vi "Diagnostics - Tool.vi"() -> ()   [LabVIEW 2019, in "Diagnostics Workspace Tool.lvlib"]
uses:
  Diagnostics Workspace Tool.lvlib
  Addon/Addon Shared/Types/Command.New.ctl
  NationalInstruments.VeriStand.SystemStorage
  SubModules/CAN-Streaming-Support/Addon/Addon Shared/Types/Direction Filter.ctl
  SubModules/CAN-Streaming-Support/Addon/Addon Shared/Types/Type Filter.ctl
  Workspace Shared/Types/Workspace.State.ctl
  Workspace Shared/Types/UI.Refs.ctl
  <vilib>/NI VeriStand/Display Template Support/DisplayTemplateSupport.llb/enum_Display Template Handler Minimal To Workspace.ctl
  Workspace Shared/Types/Workspace.SavedState.ctl
  <vilib>/NI VeriStand/Execution/Workspace/WorkspaceAPI.ctl
  <vilib>/NI VeriStand/Display Template Support/DisplayTemplateSupport.llb/enum_Display Template Handler Minimal To Widget Msg.ctl
  <vilib>/NI VeriStand/Execution/Workspace/SystemStateRegEventRef.ctl
  <vilib>/NI VeriStand/Execution/Workspace/Target State Info.ctl
  <vilib>/NI VeriStand/Execution/Workspace/Target State.ctl
  <vilib>/NI VeriStand/Execution/Workspace/SystemStateEventRef.ctl
  Addon/Addon Shared/Types/Protocol.ctl
  SubModules/CAN-Streaming-Support/UIs/Workspace Shared/Types/Host Stream Queue Refs.ctl
  SubModules/CAN-Streaming-Support/UIs/Workspace Shared/Types/Host Stream Queue Type.ctl
  SubModules/CAN-Streaming-Support/UIs/Workspace Shared/Types/Host Stream Queue Command.ctl
  <vilib>/xnet/xnet.llb/XNET Frame CAN.ctl
  <vilib>/xnet/xnet.llb/XNET Frame Type CAN.ctl
  SubModules/CAN-Streaming-Support/UIs/Workspace Shared/Types/Host Stream Engine Parameters.ctl
  SubModules/CAN-Streaming-Support/Addon/Addon Shared/Types/Filter Parameters.ctl
  Addon/Addon Shared/Types/Command.ReadDTC.ctl
  Addon/Addon Shared/Types/DTC.Descriptor.Override.ctl
  <vilib>/Utility/miscctls.llb/LVRowAndColumnUnsignedTypeDef.ctl
  <vilib>/dlg_ctls.llb/Space Constant.vi
  SubModules/CAN-Streaming-Support/UIs/Workspace Shared/SubVIs/Create Host Stream Refs.vi
  SubModules/CAN-Streaming-Support/UIs/Workspace Shared/SubVIs/Read Host Stream.vi
  SubModules/CAN-Streaming-Support/UIs/Workspace Shared/SubVIs/Cleanup Host Stream.vi
  SubModules/CAN-Streaming-Support/UIs/Workspace Shared/SubVIs/Create Bus Log File.vi
  SubModules/CAN-Streaming-Support/UIs/Workspace Shared/SubVIs/Write to Bus Log File.vi
  SubModules/CAN-Streaming-Support/UIs/Workspace Shared/SubVIs/Convert BIN to TXT File.vi
  SubModules/CAN-Streaming-Support/UIs/Workspace Shared/SubVIs/Get Next Bus Engine State.vi
  SubModules/CAN-Streaming-Support/UIs/Workspace Shared/SubVIs/Get Engine Trigger State.vi
  SubModules/CAN-Streaming-Support/UIs/Workspace Shared/SubVIs/Get Next Log Engine State.vi
  SubModules/CAN-Streaming-Support/UIs/Workspace Shared/SubVIs/Process CAN Data.vi
  SubModules/CAN-Streaming-Support/UIs/Workspace Shared/SubVIs/Process CAN State.vi
  SubModules/CAN-Streaming-Support/UIs/Workspace Shared/SubVIs/Convert Frame Array to String Array.vi
  SubModules/CAN-Streaming-Support/UIs/Workspace Shared/SubVIs/Convert Time to UTC String.vi
  <userlib>/_OpenG.lib/array/array.llb/Sort Array__ogtk.vi
  <userlib>/_OpenG.lib/array/array.llb/Sort 2D Array (String)__ogtk.vi
  <vilib>/Utility/libraryn.llb/Check if File or Folder Exists.vi
  <vilib>/Utility/libraryn.llb/Get File Extension.vi
  Addon/Addon Shared/SubVIs/Constants.vi
  <vilib>/NI VeriStand/Execution/Workspace/NI VeriStand - Get Multiple Channel Values.vi
  <vilib>/NI VeriStand/Execution/Workspace/NI VeriStand - Set Single Channel Value.vi
  Workspace Shared/Diagnostics Workspace Shared.lvlib
  APIs/Host Automation API/Diagnostics Host Automation API.lvlib
  Addon/Addon Shared/Diagnostics Addon Shared.lvlib
  <vilib>/NI VeriStand/Execution/Workspace/NI_VS Workspace ExecutionAPI.lvlib
  SubModules/CAN-Streaming-Support/UIs/Workspace Shared/CAN Stream Support Workspace Shared.lvlib
  SubModules/CAN-Streaming-Support/Addon/Addon Shared/CAN Stream Support Shared.lvlib
  NationalInstruments.VeriStand.ClientAPI
panel:
  out "Device":string
  in  "Tab Control":enum32{"Cmd", "Raw", "Read DTCs", "Bus Stream"}(tab)
  out "Time Stamp":timestamp
  out "CAN Connected?":bool
  in  "Send Cmd":bool
  out "VeriStand Error":i64 format="%.0x"
  out "Success?":bool
  in  "Cmd":T1
  in  "Clear Raw":bool
  in  "Send Raw":bool
  out "Raw VeriStand Error":errorcluster
  out "Raw Error Byte":u8 format="%.0x"
  in  "Response Required?":bool
  out "Raw Resp":u8[](array[numeric]) format="%.0x"
  in  "Raw Cmd":u8[](array[numeric]) format="%.0x"
  in  "DTC":u32
  in  "Status":u32
  in  "Failure":u32
  in  "Override Byte Lengths":bool
  in  "Extension":u32 format="%.0x"
  in  "Mask":u32 format="%.0x"
  in  "Mode":u32 format="%.0x"
  in  "Hex":bool=TRUE
  in  "DTCs":string(tree)
  in  "Read DTCs":bool
  in  "Reset Filter":bool
  in  "Host Filter":bool
  in  "Filter IDs":string caption="Filter IDs (format = x<ID>, comma seperated, ID x0 = Bus Error)"
  in  "Clear History":bool
  in  "Type Filter":T2
  out "Table Control":string[][](table)
  in  "Enable Stream":bool
  in  "Pause":bool
  in  "Sort By ID":bool
  out "Stream Connected":bool
  out "Status":string
  in  "Direction Filter":T3
  in  "Log":bool
  in  "NIVS.Gateway IP Address":string
  in  "NIVS.System Definition Root":refnum<k24>
  in  "NIVS.Workspace Event":refnum<event-registration>
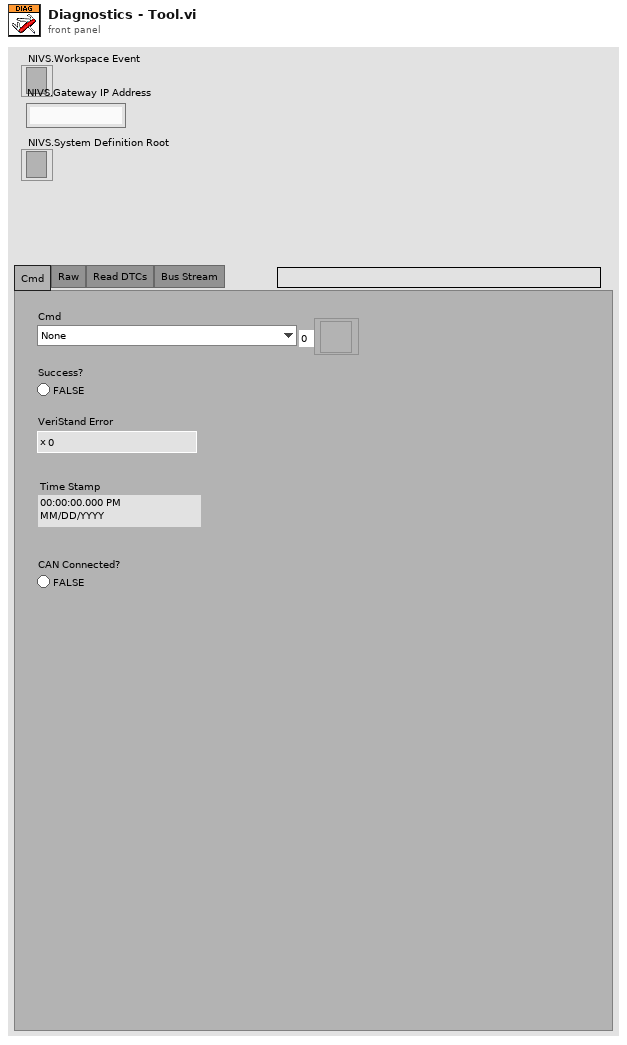
[diagram p1: front panel]
types:
  T1 = typedef "Diagnostics Addon Shared.lvlib/Command.New.ctl" = enum8{"None", "Clear Status Channels", "Read All DIDs", "Read All PIDs", "Configure and Start DPIDs", "Stop DPIDs"}
  T2 = typedef "CAN Stream Support Shared.lvlib/Type Filter.ctl" = enum16{"All", "CAN Data", "CAN Remote", "CAN Bus Error", "CAN 2.0 Data", "CAN FD Data", "CAN FD+BRS Data", "J1939 Data", "Delay", "Log Trigger", "Start Trigger"}
  T3 = typedef "CAN Stream Support Shared.lvlib/Direction Filter.ctl" = enum16{"Tx/Rx", "Rx", "Tx"}
  T4 = typedef "Diagnostics Workspace Shared.lvlib/Workspace.State.ctl" = cluster{"UI.Refs":T5, "Data.PreviousValues":dbl[], "Data.Read":string[], "CachedData.UserEvent":refnum<user-event>, "CachedData":T6, "Addon.Connected?":bool, "NIVS.SysDef":path, "NIVS.SysDefRoot":refnum<k24>, "NIVS.Workspace":T7, "NIVS.UserEventRefs":cluster{"Event Registration Refnum":refnum<event-registration>, "SystemChangeEventRef":T8, "NIVS.Workspace Event":refnum<event-registration>}, "NIVS.SystemStateRefs":T9, "NIVS.LaunchRef":refnum<user-event>, "Data.PendingChange?":bool, "Command.Channel":string, "Diagnostic Protocol":T10, "Channels.Found":bool, "Command.Connect":string, "Mode.Tool?":bool, "Stream.Qs":T11}
  T5 = typedef "Diagnostics Workspace Shared.lvlib/UI.Refs.ctl" = cluster{"Cmd":refnum<vi>, "Success?":refnum<vi>, "VeriStandError":refnum<vi>, "CAN Connected?":refnum<vi>, "DTC":refnum<vi>, "Status":refnum<vi>, "Failure":refnum<vi>, "Override Byte Lengths":refnum<vi>, "Response Required?":refnum<vi>, "Send":refnum<vi>, "Clear":refnum<vi>, "Send Raw":refnum<vi>, "Read DTCs":refnum<vi>, "Raw Cmd":refnum<vi>, "Extension":refnum<vi>, "Mode":refnum<vi>, "Mask":refnum<vi>, "Hex":refnum<vi>, "Raw Resp":refnum<vi>, "Raw Error Byte":refnum<vi>, "Raw VeriStand Error":refnum<vi>, "DTCs":refnum<vi>, "Time Stamp":refnum<vi>, "Device":refnum<vi>, "Pause":refnum<vi>, "Table Control":refnum<vi>, "Sort By ID":refnum<vi>, "Streaming Connected":refnum<vi>, "Enable Stream":refnum<vi>, "CAN State":refnum<vi>, "Direction Filter":refnum<vi>, "Type Filter":refnum<vi>, "Clear History":refnum<vi>, "Filter IDs":refnum<vi>, "Filter Location":refnum<vi>, "Reset Filter":refnum<vi>, "Log":refnum<vi>}
  T6 = typedef "Diagnostics Workspace Shared.lvlib/Workspace.SavedState.ctl" = cluster{"CD Path":string, "CD IP":string}
  T7 = typedef "NI_VS Workspace ExecutionAPI.lvlib/WorkspaceAPI.ctl" = refnum<k24>
  T8 = typedef "NI_VS Workspace ExecutionAPI.lvlib/SystemStateRegEventRef.ctl" = refnum<event-registration>
  T9 = typedef "NI_VS Workspace ExecutionAPI.lvlib/SystemStateEventRef.ctl" = cluster{"CustDatRef":refnum<user-event>, "EvtRef":refnum<k27>, "Target State User Event":refnum<user-event>}
  T10 = typedef "Diagnostics Addon Shared.lvlib/Protocol.ctl" = enum16{"GMLAN", "KWP-2000", "UDS", "User-Defined"}
  T11 = typedef "CAN Stream Support Workspace Shared.lvlib/Host Stream Queue Refs.ctl" = cluster{"Cmd Q":refnum<queue>, "XNET Frames":refnum<queue>}
  T12 = typedef "enum_Display Template Handler Minimal To Workspace.ctl" = cluster{"Operation":enum16{"SetCustomData", "DeleteItem"}, "Data":variant}
  T13 = typedef "Diagnostics Addon Shared.lvlib/Command.ReadDTC.ctl" = cluster{"Extension":u32, "Mask":u32, "Mode/Status":u32, "Byte Lengths":T14}
  T14 = typedef "Diagnostics Addon Shared.lvlib/DTC.Descriptor.Override.ctl" = cluster{"Override":bool, "DTC":u32, "Status":u32, "Failure":u32}
  T15 = typedef "CAN Stream Support Shared.lvlib/Filter Parameters.ctl" = cluster{"ID Filters":u32[], "Direction Filter":T3, "Type Filter":T2}
  T16 = typedef "LVRowAndColumnUnsignedTypeDef.ctl" = cluster{"Row":u32, "Column":u32}
  T17 = cluster{"Event Registration Refnum":refnum<event-registration>, "SystemChangeEventRef":T8, "NIVS.Workspace Event":refnum<event-registration>}
  T18 = typedef "enum_Display Template Handler Minimal To Widget Msg.ctl" = enum16{"Stop", "LaunchConfigDialog"}
  T19 = typedef "Diagnostics Addon Shared.lvlib/UI.Refs.ctl" = cluster{"Cmd":refnum<vi>, "Success?":refnum<vi>, "VeriStandError":refnum<vi>, "CAN Connected?":refnum<vi>, "DTC":refnum<vi>, "Status":refnum<vi>, "Failure":refnum<vi>, "Override Byte Lengths":refnum<vi>, "Response Required?":refnum<vi>, "Send":refnum<vi>, "Clear":refnum<vi>, "Send Raw":refnum<vi>, "Read DTCs":refnum<vi>, "Raw Cmd":refnum<vi>, "Extension":refnum<vi>, "Mode":refnum<vi>, "Mask":refnum<vi>, "Hex":refnum<vi>, "Raw Resp":refnum<vi>, "Raw Error Byte":refnum<vi>, "Raw VeriStand Error":refnum<vi>, "DTCs":refnum<vi>, "Time Stamp":refnum<vi>, "Device":refnum<vi>, "Pause":refnum<vi>, "Table Control":refnum<vi>, "Sort By ID":refnum<vi>, "Streaming Connected":refnum<vi>, "Enable Stream":refnum<vi>, "CAN State":refnum<vi>, "Direction Filter":refnum<vi>, "Type Filter":refnum<vi>, "Clear History":refnum<vi>, "Filter IDs":refnum<vi>, "Filter Location":refnum<vi>, "Reset Filter":refnum<vi>, "Log":refnum<vi>}
  T20 = enum8{"Enabled", "Disabled", "Disabled and Grayed Out"}
  T21 = typedef "Diagnostics Addon Shared.lvlib/HostAutomation.Ref.ctl" = cluster{"TCP Comm":T22, "DTCs":T24}
  T22 = typedef "NI STM.lvlib/TCP Connection Info.ctl" = cluster{"connection ID":refnum<k5>, "meta data":T23[]}
  T23 = typedef "NI STM.lvlib/MetaDataElement.ctl" = string
  T24 = typedef "Diagnostics Addon Shared.lvlib/DTC.Codes.ctl" = cluster{"Value.Code":dbl[], "Value.String":string[], "Value.J2012String":string[], "Status.Code":dbl[], "Status.String":string[]}
  T25 = cluster{"resp":u8[], "error code":u8, "error out":errorcluster}
  T26 = typedef "Diagnostics Addon Shared.lvlib/Command.ReadDTC.DTCs.ctl" = cluster{"Timestamp":dbl, "DTC":dbl, "J2012 String":string, "DTC String":string, "Status":dbl, "Status String":string, "Add Data":dbl}
  T27 = typedef "CAN Stream Support Workspace Shared.lvlib/Host Stream Engine Parameters.ctl" = cluster{"Host Filter":bool, "Filter Parameters":T15, "Sort By ID":bool, "Pause":bool, "Clear History":bool, "Log":bool}
  T28 = typedef "CAN Stream Support Workspace Shared.lvlib/Host Stream Data.ctl" = cluster{"Connected":bool, "Bus Data Update":bool, "Bus Data":string[][], "Bus Status":string, "Bus Warning":bool, "Log Status":string}
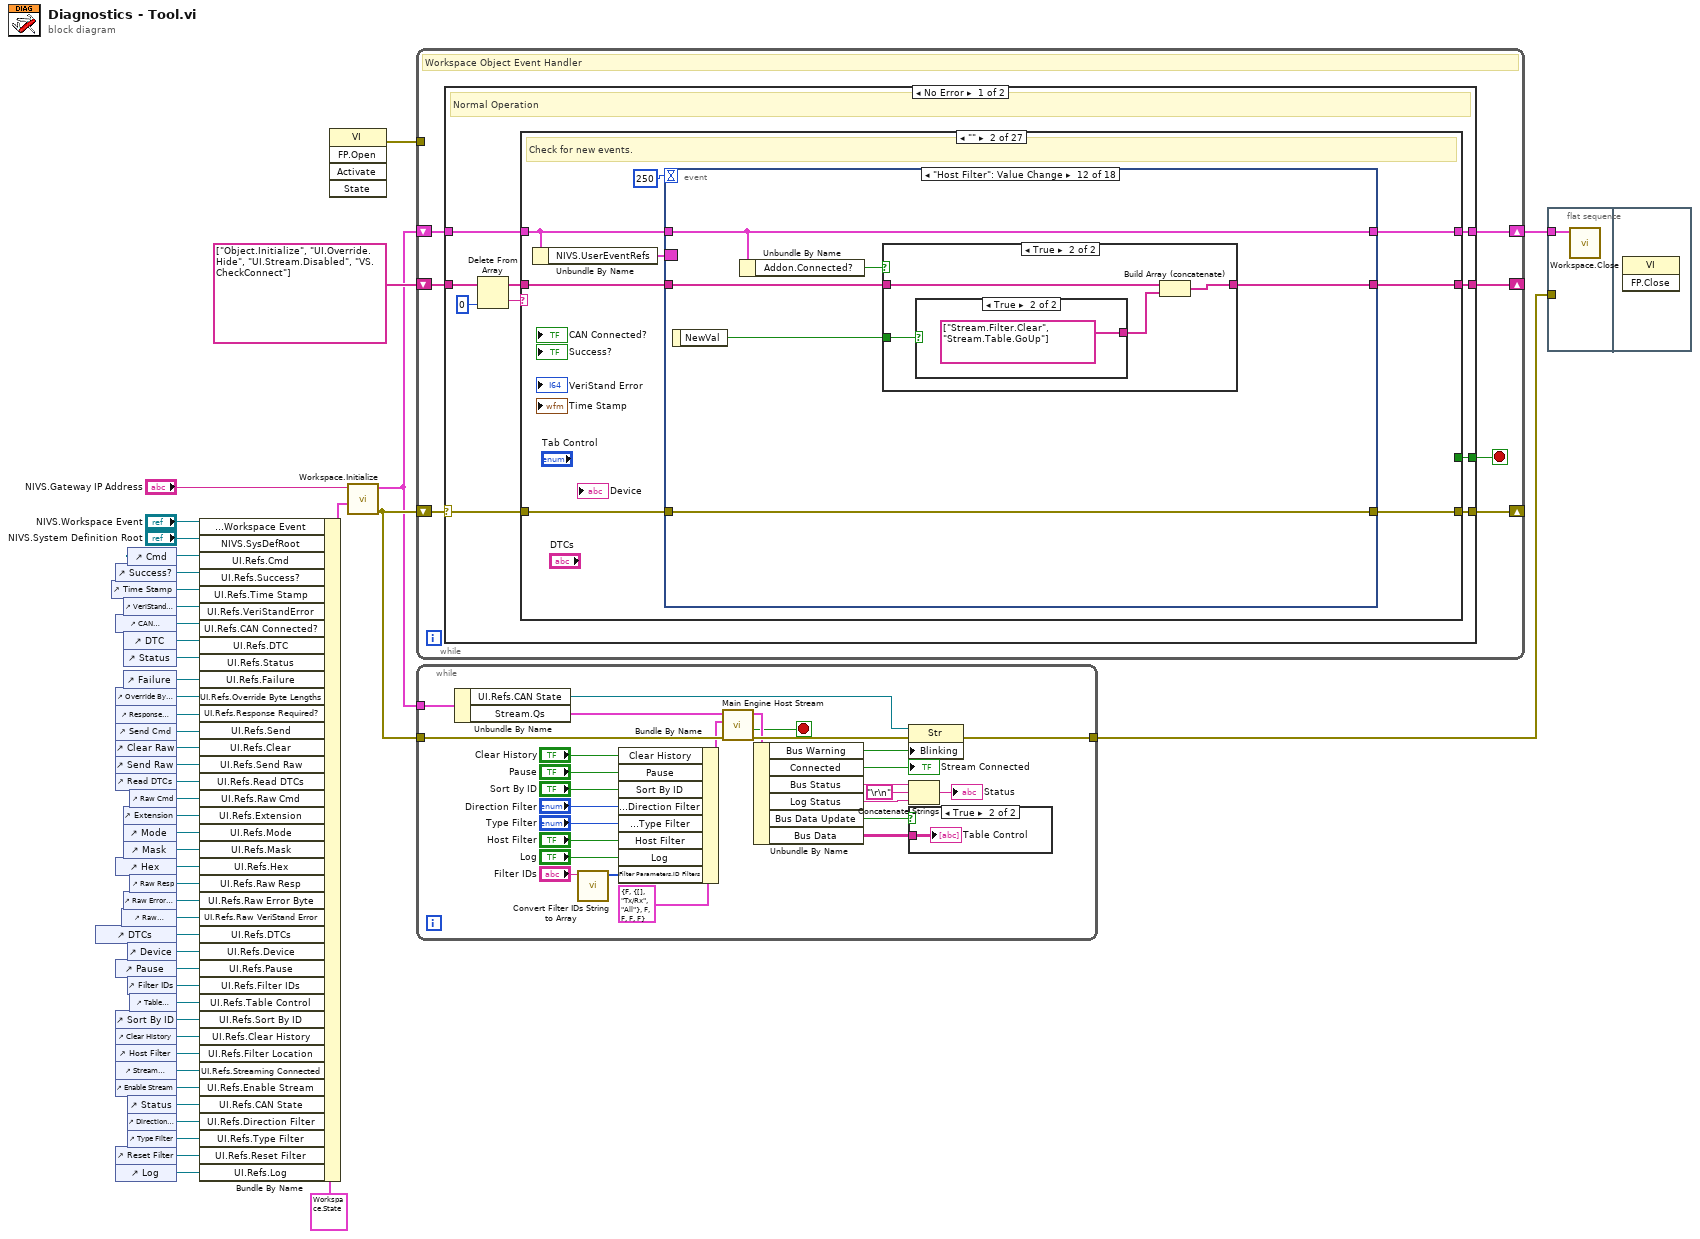
[diagram p0: block diagram]
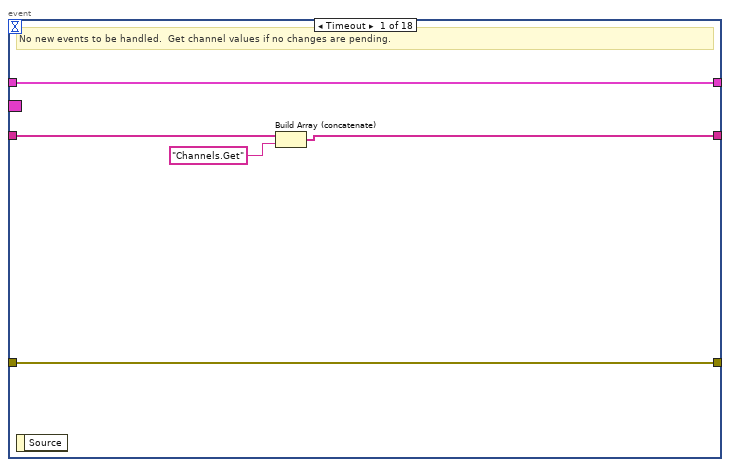
[diagram p4: hidden frame]
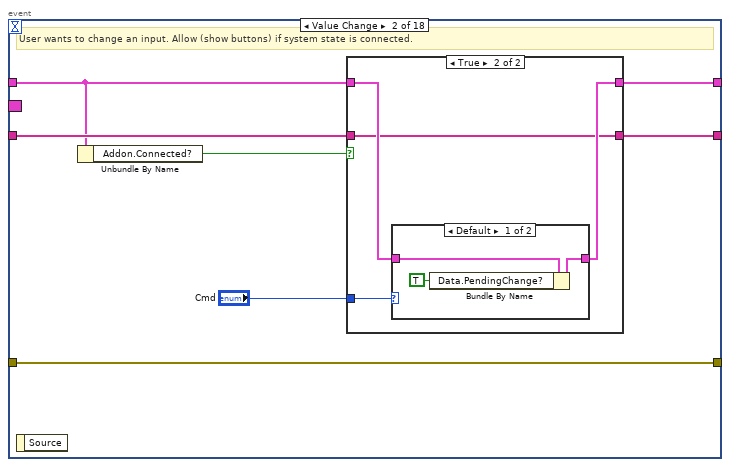
[diagram p5: hidden frame]
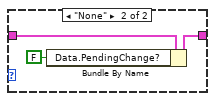
[diagram p7: hidden frame]
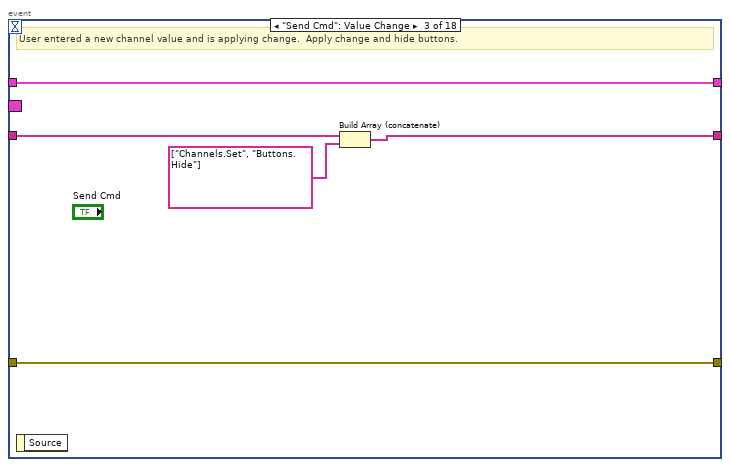
[diagram p8: hidden frame]
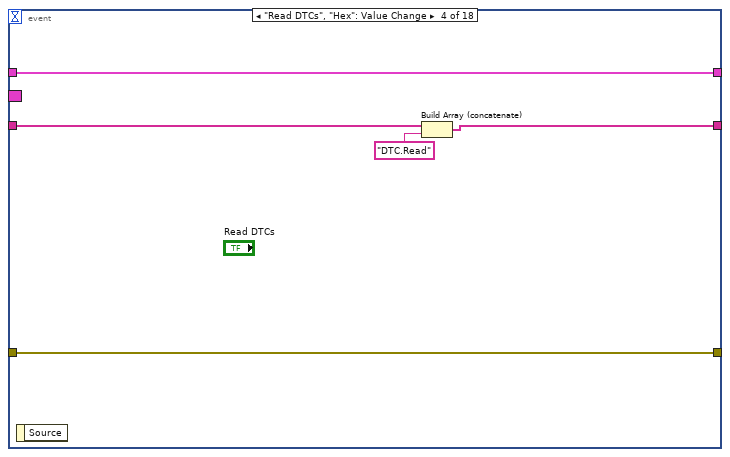
[diagram p9: hidden frame]
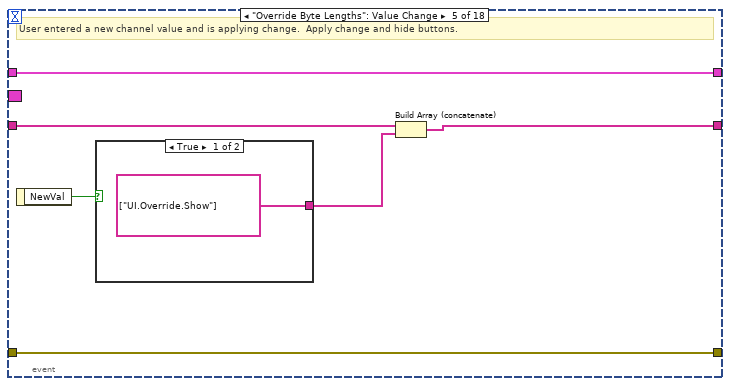
[diagram p10: hidden frame]
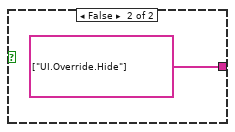
[diagram p11: hidden frame]
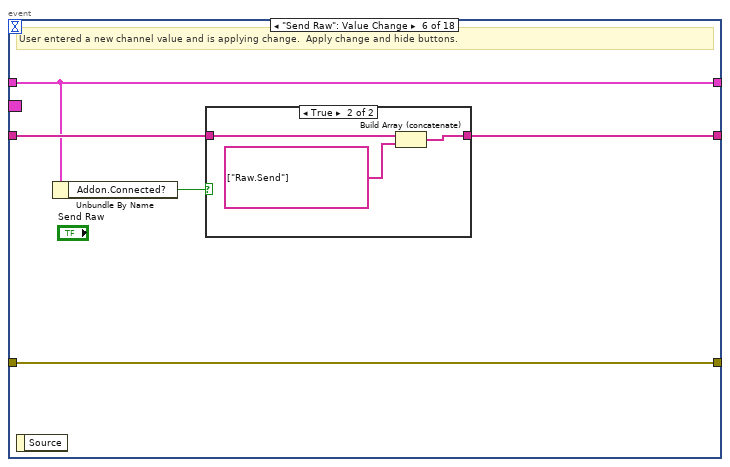
[diagram p12: hidden frame]
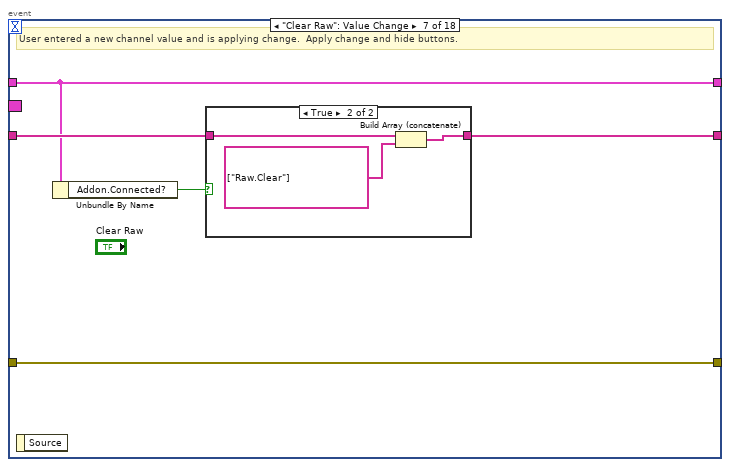
[diagram p14: hidden frame]
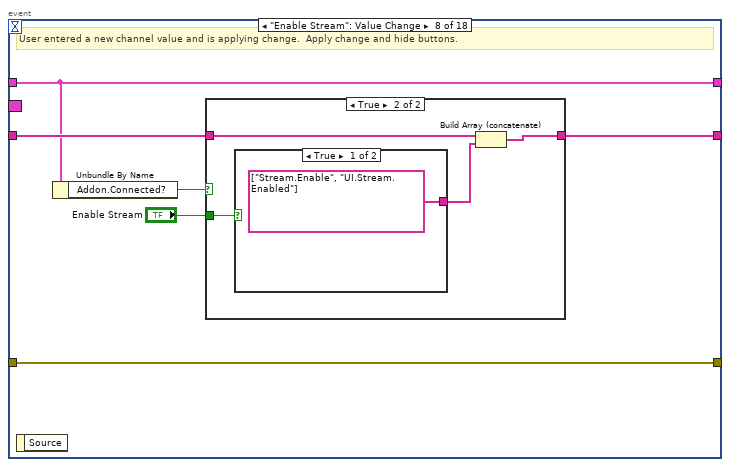
[diagram p16: hidden frame]
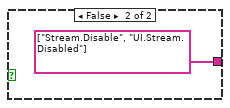
[diagram p18: hidden frame]
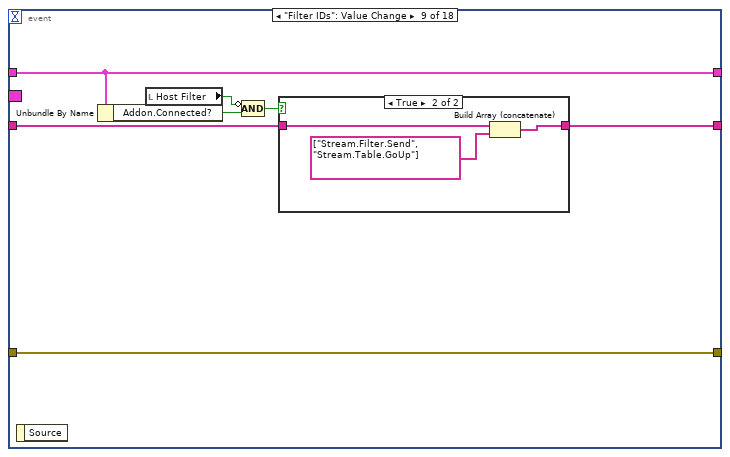
[diagram p19: hidden frame]
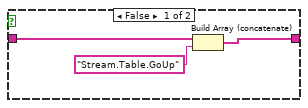
[diagram p20: hidden frame]
diagram:
  n1 = control-ref of="DTCs"() -> (w23:refnum<vi>)
  n2 = control-ref of="Time Stamp"() -> (w18:refnum<vi>)
  n3 = control-ref of="Success?"() -> (w44:refnum<vi>)
  n4 = control-ref of="CAN Connected?"() -> (w43:refnum<vi>)
  n5 = control-ref of="Override Byte Lengths"() -> (w39:refnum<vi>)
  n6 = control-ref of="Response Required?"() -> (w33:refnum<vi>)
  n7 = control-ref of="Send Cmd"() -> (w32:refnum<vi>)
  n8 = control-ref of="Clear Raw"() -> (w31:refnum<vi>)
  n9 = control-ref of="Send Raw"() -> (w30:refnum<vi>)
  n10 = control-ref of="Read DTCs"() -> (w29:refnum<vi>)
  n11 = control-ref of="Hex"() -> (w24:refnum<vi>)
  n12 = control-ref of="Pause"() -> (w16:refnum<vi>)
  n13 = control-ref of="Sort By ID"() -> (w14:refnum<vi>)
  n14 = control-ref of="Clear History"() -> (w4:refnum<vi>)
  n15 = control-ref of="Host Filter"() -> (w3:refnum<vi>)
  n16 = control-ref of="Stream Connected"() -> (w13:refnum<vi>)
  n17 = control-ref of="Enable Stream"() -> (w12:refnum<vi>)
  n18 = control-ref of="Reset Filter"() -> (w2:refnum<vi>)
  n19 = control-ref of="Log"() -> (w1:refnum<vi>)
  n20 = control-ref of="Raw VeriStand Error"() -> (w22:refnum<vi>)
  n21 = control-ref of="VeriStand Error"() -> (w45:refnum<vi>)
  n22 = control-ref of="DTC"() -> (w42:refnum<vi>)
  n23 = control-ref of="Status"() -> (w41:refnum<vi>)
  n24 = control-ref of="Failure"() -> (w40:refnum<vi>)
  n25 = control-ref of="Extension"() -> (w27:refnum<vi>)
  n26 = control-ref of="Mode"() -> (w26:refnum<vi>)
  n27 = control-ref of="Mask"() -> (w25:refnum<vi>)
  n28 = control-ref of="Raw Error Byte"() -> (w21:refnum<vi>)
  n29 = control-ref of="Cmd"() -> (w19:refnum<vi>)
  n30 = control-ref of="Device"() -> (w17:refnum<vi>)
  n31 = control-ref of="Filter IDs"() -> (w5:refnum<vi>)
  n32 = control-ref of="Status"() -> (w11:refnum<vi>)
  n33 = control-ref of="Direction Filter"() -> (w7:refnum<vi>)
  n34 = control-ref of="Type Filter"() -> (w6:refnum<vi>)
  n35 = control-ref of="Raw Cmd"() -> (w28:refnum<vi>)
  n36 = control-ref of="Raw Resp"() -> (w20:refnum<vi>)
  n37 = control-ref of="Table Control"() -> (w15:refnum<vi>)
  n38 = Bundle By Name(cluster=T4 {"UI.Refs"={"Cmd"=refnum, "Success?"=refnum, "VeriStandError"=refnum, "CAN Connected?"=refnum, "DTC"=refnum, "Status"=refnum, "Failure"=refnum, "Override Byte Lengths"=refnum, "Response Required?"=refnum, "Send"=refnum, "Clear"=refnum, "Send Raw"=refnum, "Read DTCs"=refnum, "Raw Cmd"=refnum, "Extension"=refnum, "Mode"=refnum, "Mask"=refnum, "Hex"=refnum, "Raw Resp"=refnum, "Raw Error Byte"=refnum, "Raw VeriStand Error"=refnum, "DTCs"=refnum, "Time Stamp"=refnum, "Device"=refnum, "Pause"=refnum, "Table Control"=refnum, "Sort By ID"=refnum, "Streaming Connected"=refnum, "Enable Stream"=refnum, "CAN State"=refnum, "Direction Filter"=refnum, "Type Filter"=refnum, "Clear History"=refnum, "Filter IDs"=refnum, "Filter Location"=refnum, "Reset Filter"=refnum, "Log"=refnum}, "Data.PreviousValues"=[], "Data.Read"=[], "CachedData.UserEvent"=refnum, "CachedData"={"CD Path"="", "CD IP"=""}, "Addon.Connected?"=FALSE, "NIVS.SysDef"=path "", "NIVS.SysDefRoot"=refnum, "NIVS.Workspace"=refnum, "NIVS.UserEventRefs"={"Event Registration Refnum"=refnum, "SystemChangeEventRef"=refnum, "NIVS.Workspace Event"=refnum}, "NIVS.SystemStateRefs"={"CustDatRef"=refnum, "EvtRef"=refnum, "Target State User Event"=refnum}, "NIVS.LaunchRef"=refnum, "Data.PendingChange?"=FALSE, "Command.Channel"="", "Diagnostic Protocol"=enum."GMLAN", "Channels.Found"=FALSE, "Command.Connect"="", "Mode.Tool?"=FALSE, "Stream.Qs"={"Cmd Q"=refnum, "XNET Frames"=refnum}}, "NIVS.UserEventRefs.NIVS.Workspace Event"="NIVS.Workspace Event", "NIVS.SysDefRoot"="NIVS.System Definition Root", "UI.Refs.Cmd"=w19, "UI.Refs.Success?"=w44, "UI.Refs.Time Stamp"=w18, "UI.Refs.VeriStandError"=w45, "UI.Refs.CAN Connected?"=w43, "UI.Refs.DTC"=w42, "UI.Refs.Status"=w41, "UI.Refs.Failure"=w40, "UI.Refs.Override Byte Lengths"=w39, "UI.Refs.Response Required?"=w33, "UI.Refs.Send"=w32, "UI.Refs.Clear"=w31, "UI.Refs.Send Raw"=w30, "UI.Refs.Read DTCs"=w29, "UI.Refs.Raw Cmd"=w28, "UI.Refs.Extension"=w27, "UI.Refs.Mode"=w26, "UI.Refs.Mask"=w25, "UI.Refs.Hex"=w24, "UI.Refs.Raw Resp"=w20, "UI.Refs.Raw Error Byte"=w21, "UI.Refs.Raw VeriStand Error"=w22, "UI.Refs.DTCs"=w23, "UI.Refs.Device"=w17, "UI.Refs.Pause"=w16, "UI.Refs.Filter IDs"=w5, "UI.Refs.Table Control"=w15, "UI.Refs.Sort By ID"=w14, "UI.Refs.Clear History"=w4, "UI.Refs.Filter Location"=w3, "UI.Refs.Streaming Connected"=w13, "UI.Refs.Enable Stream"=w12, "UI.Refs.CAN State"=w11, "UI.Refs.Direction Filter"=w7, "UI.Refs.Type Filter"=w6, "UI.Refs.Reset Filter"=w2, "UI.Refs.Log"=w1) -> (w46:T4)
  n39 = invoke class="VI" method="FP.Open"() -> (error out=w37:errorcluster)  [unwired: 5 in, 4 out]
  n40 = call "Workspace.Initialize.vi"("State Variables in"=w46, "NIVS.Gateway IP Address"="NIVS.Gateway IP Address") -> ("error out"=w10:errorcluster, "State Variables out"=w9:T4)  [unwired: 8 in]
  n41 = while {
    shift-right: [w53] -> _
    shift-left: string[] ["Object.Initialize", "UI.Override.Hide", "UI.Stream.Disabled", "VS.CheckConnect"] -> [w54]
    shift-right: [w51] -> w36
    shift-left: w9 -> [w50]
    shift-right: [w52] -> _
    shift-left: w10 -> [w49]
    tunnel: w37 -> [_]
    stop <- w55 stop-if-true
    # "Workspace Object Event Handler"
    n42 = case shown="No Error" w49 {
      selector: w49 -> [w56 w619]
      tunnel: [w65 _] -> w55
      tunnel: w54 -> [w63 w626]
      tunnel: [w60 w626] -> w53
      tunnel: [w59 w617] -> w52
      tunnel: [w58 w625] -> w51
      tunnel: w50 -> [w57 w625]
      frame No Error {
        # "Normal Operation"
        n43 = Delete From Array(array=w63, index=0) -> (deleted portion=w62:string, array with subset deleted=w61:string[])  [unwired: 1 in]
        n44 = case shown="\"\"" w62 {
          tunnel: [_ _ _ _ _ _ _ TRUE _ _ _ _ _ _ _ _ _ _ _ _ _ _ _ _ _ _ _] -> w65
          tunnel: [w68 w75 w270 w277 w312 w329 w335 w356 w363 w376 w399 w417 w430 w438 w452 w465 w478 w501 w505 w530 w539 w557 w569 w586 w605 w611 w616] -> w60
          tunnel: w56 -> [w67 w73 w271 w283 w308 w327 w340 w353 w362 w374 w398 w411 w424 w436 w449 w463 w475 w500 w504 w509 w538 w550 w562 w579 w596 w606 w612]
          tunnel: w61 -> [w68 w74 w270 w276 w312 w329 w334 w356 w363 w376 w399 w417 w430 w438 w452 w465 w478 w501 w505 w530 w539 w557 w569 w586 w605 w611 w616]
          tunnel: w57 -> [w66 w69 w267 w281 w313 w326 w332 w352 w359 w369 w396 w416 w429 w435 w451 w464 w477 w497 w503 w529 w536 w553 w565 w582 w599 w610 w615]
          tunnel: [w67 w72 w263 w283 w297 w324 w339 w354 w362 w373 w397 w410 w423 w437 w440 w462 w467 w500 w504 w507 w537 w550 w562 w579 w596 w607 w613] -> w59
          tunnel: [w66 w71 w267 w280 w295 w325 w333 w352 w359 w372 w395 w416 w429 w435 w451 w464 w477 w497 w503 w529 w536 w553 w565 w582 w599 w610 w615] -> w58
          frame Default {
            # "Do nothing."
          }
          frame "" {
            # "Check for new events."
            n45 = Unbundle By Name(w69) -> ("NIVS.UserEventRefs"=w70:T17)
            n46 = event shown="[11] \"Host Filter\": Value Change" {
              selector: w70 -> [_ _ _ _ _ _ _ _ _ _ _ _ _ _ _ _ _ _]
              dyn-events: _ -> [_ _ _ _ _ _ _ _ _ _ _ _ _ _ _ _ _ _]
              timeout: 250 -> [_ _ _ _ _ _ _ _ _ _ _ _ _ _ _ _ _ _]
              tunnel: [w77 w86 w101 w106 w114 w121 w130 w140 w155 w166 w175 w185 w198 w208 w221 w237 w251 w258] -> w75
              tunnel: w74 -> [w80 w87 w102 w107 w115 w122 w131 w141 w154 w165 w174 w184 w197 w210 w220 w236 w252 w259]
              tunnel: w73 -> [w81 w82 w105 w110 w116 w123 w132 w142 w156 w167 w176 w186 w199 w207 w228 w235 w255 w261]
              tunnel: [w81 w82 w105 w110 w116 w123 w132 w142 w156 w167 w176 w186 w199 w207 w228 w235 w255 w261] -> w72
              tunnel: [w78 w88 w104 w109 w113 w120 w129 w139 w153 w164 w173 w183 w196 w212 w227 w233 w254 w260] -> w71
              tunnel: w69 -> [w78 w85 w104 w109 w113 w120 w129 w139 w153 w164 w173 w183 w196 w212 w227 w234 w254 w260]
              event Timeout {
                # "No new events to be handled.  Get channel values if no changes are pending."
                n47 = event-data() -> ()  [unwired: 2 out]
                n48 = Build Array (concatenate)(w80, "Channels.Get") -> (w77:string[])
              }
              event Value Change {
                # "User wants to change an input. Allow (show buttons) if system state is connected."
                n49 = event-data() -> ()  [unwired: 2 out]
                n50 = Unbundle By Name(w85) -> ("Addon.Connected?"=w84:bool)
                n51 = case shown="True" w84 {
                  tunnel: w85 -> [w89 w94]
                  tunnel: [w89 w93] -> w88
                  tunnel: w87 -> [w90 w92]
                  tunnel: [w90 w92] -> w86
                  tunnel: "Cmd" -> [_ w91]
                  frame False {
                  }
                  frame True {
                    n52 = case shown="Default" w91 {
                      tunnel: w94 -> [w96 w99]
                      tunnel: [w95 w98] -> w93
                      frame Default {
                        n53 = Bundle By Name(cluster=w96, "Data.PendingChange?"=TRUE ("Pending Change?")) -> (w95:T4)
                      }
                      frame "None" {
                        n54 = Bundle By Name(cluster=w99, "Data.PendingChange?"=FALSE ("Pending Change?")) -> (w98:T4)
                      }
                    }
                  }
                }
              }
              event "Send Cmd": Value Change {
                # "User entered a new channel value and is applying change.  Apply change and hide buttons."
                n55 = event-data() -> ()  [unwired: 2 out]
                n56 = Build Array (concatenate)(w102, string[] ["Channels.Set", "Buttons.Hide"]) -> (w101:string[])
              }
              event "Read DTCs", "Hex": Value Change {
                n57 = event-data() -> ()  [unwired: 2 out]
                n58 = Build Array (concatenate)(w107, "DTC.Read") -> (w106:string[])
              }
              event "Override Byte Lengths": Value Change {
                # "User entered a new channel value and is applying change.  Apply change and hide buttons."
                n59 = event-data() -> ("NewVal"=w111:bool)  [unwired: 1 out]
                n60 = case shown="True" w111 {
                  tunnel: [string[] ["UI.Override.Show"] string[] ["UI.Override.Hide"]] -> w112
                  frame True {
                  }
                  frame False {
                  }
                }
                n61 = Build Array (concatenate)(w115, w112) -> (w114:string[])
              }
              event "Send Raw": Value Change {
                # "User entered a new channel value and is applying change.  Apply change and hide buttons."
                n62 = event-data() -> ()  [unwired: 2 out]
                n63 = Unbundle By Name(w120) -> ("Addon.Connected?"=w119:bool)
                n64 = case shown="True" w119 {
                  tunnel: w122 -> [w124 w126]
                  tunnel: [w124 w125] -> w121
                  frame False {
                  }
                  frame True {
                    n65 = Build Array (concatenate)(w126, string[] ["Raw.Send"]) -> (w125:string[])
                  }
                }
              }
              event "Clear Raw": Value Change {
                # "User entered a new channel value and is applying change.  Apply change and hide buttons."
                n66 = event-data() -> ()  [unwired: 2 out]
                n67 = Unbundle By Name(w129) -> ("Addon.Connected?"=w128:bool)
                n68 = case shown="True" w128 {
                  tunnel: w131 -> [w133 w135]
                  tunnel: [w133 w134] -> w130
                  frame False {
                  }
                  frame True {
                    n69 = Build Array (concatenate)(w135, string[] ["Raw.Clear"]) -> (w134:string[])
                  }
                }
              }
              event "Enable Stream": Value Change {
                # "User entered a new channel value and is applying change.  Apply change and hide buttons."
                n70 = event-data() -> ()  [unwired: 2 out]
                n71 = Unbundle By Name(w139) -> ("Addon.Connected?"=w138:bool)
                n72 = case shown="True" w138 {
                  tunnel: w141 -> [w143 w146]
                  tunnel: [w143 w145] -> w140
                  tunnel: "Enable Stream" -> [_ w144]
                  frame False {
                  }
                  frame True {
                    n73 = case shown="True" w144 {
                      tunnel: [string[] ["Stream.Enable", "UI.Stream.Enabled"] string[] ["Stream.Disable", "UI.Stream.Disabled"]] -> w147
                      frame True {
                      }
                      frame False {
                      }
                    }
                    n74 = Build Array (concatenate)(w146, w147) -> (w145:string[])
                  }
                }
              }
              event "Filter IDs": Value Change {
                n75 = event-data() -> ()  [unwired: 2 out]
                n76 = Unbundle By Name(w153) -> ("Addon.Connected?"=w151:bool)
                n77 = local read "Host Filter"() -> (w152:bool)
                n78 = Compound Arithmetic op=AND(invert w152, w151) -> (w150:bool)
                n79 = case shown="True" w150 {
                  tunnel: w154 -> [w157 w161]
                  tunnel: [w158 w160] -> w155
                  frame False {
                    n80 = Build Array (concatenate)(w157, "Stream.Table.GoUp") -> (w158:string[])
                  }
                  frame True {
                    n81 = Build Array (concatenate)(w161, string[] ["Stream.Filter.Send", "Stream.Table.GoUp"]) -> (w160:string[])
                  }
                }
              }
              event "Clear History", "Sort By ID": Value Change {
                n82 = event-data() -> ()  [unwired: 2 out]
                n83 = Unbundle By Name(w164) -> ("Addon.Connected?"=w163:bool)
                n84 = case shown="True" w163 {
                  tunnel: [w168 w171] -> w166
                  tunnel: w165 -> [w168 w170]
                  frame False {
                  }
                  frame True {
                    n85 = Build Array (concatenate)(w170, "Stream.Table.GoUp") -> (w171:string[])
                  }
                }
              }
              event "Reset Filter": Value Change {
                n86 = event-data() -> ()  [unwired: 2 out]
                n87 = Unbundle By Name(w173) -> ("Addon.Connected?"=w172:bool)
                n88 = case shown="True" w172 {
                  tunnel: w174 -> [w177 w179]
                  tunnel: [w177 w178] -> w175
                  frame False {
                  }
                  frame True {
                    n89 = Build Array (concatenate)(w179, string[] ["Stream.Filter.Reset", "Stream.Table.GoUp"]) -> (w178:string[])
                  }
                }
              }
              event "Host Filter": Value Change {
                n90 = event-data() -> ("NewVal"=w181:bool)  [unwired: 1 out]
                n91 = Unbundle By Name(w183) -> ("Addon.Connected?"=w182:bool)
                n92 = case shown="True" w182 {
                  tunnel: w184 -> [w187 w190]
                  tunnel: [w187 w189] -> w185
                  tunnel: w181 -> [_ w188]
                  frame False {
                  }
                  frame True {
                    n93 = case shown="True" w188 {
                      tunnel: [string[] ["Stream.Filter.Send", "Stream.Table.GoUp"] string[] ["Stream.Filter.Clear", "Stream.Table.GoUp"]] -> w191
                      frame False {
                      }
                      frame True {
                      }
                    }
                    n94 = Build Array (concatenate)(w190, w191) -> (w189:string[])
                  }
                }
              }
              event "Log": Value Change {
                n95 = event-data() -> ("NewVal"=w194:bool)  [unwired: 1 out]
                n96 = Unbundle By Name(w196) -> ("Addon.Connected?"=w195:bool)
                n97 = case shown="True" w195 {
                  tunnel: w197 -> [w200 w203]
                  tunnel: [w200 w202] -> w198
                  tunnel: w194 -> [_ w201]
                  frame False {
                  }
                  frame True {
                    n98 = case shown="False" w201 {
                      tunnel: [string[] ["UI.Log.Disabled"] string[] ["UI.Log.Enabled"]] -> w204
                      frame False {
                      }
                      frame True {
                      }
                    }
                    n99 = Build Array (concatenate)(w203, w204) -> (w202:string[])
                  }
                }
              }
              event User Event {
                # "System state has changed. Handle accordingly."
                n100 = event-data() -> ("SystemStateChange"=w211:string)  [unwired: 1 out]
                n101 = Unbundle By Name(w212) -> ("Mode.Tool?"=w213:bool)
                n102 = case shown="False" w213 {
                  tunnel: ["VS.CheckConnect" w216] -> w209
                  tunnel: w211 -> [_ w215]
                  frame False {
                  }
                  frame True {
                    n103 = case shown="\"Stop Configuration\"" w215 {
                      tunnel: ["Object.Exit" "VS.CheckConnect"] -> w216
                      frame "Stop Configuration" {
                      }
                      frame Default {
                      }
                    }
                  }
                }
                n104 = Build Array (concatenate)(w210, w209) -> (w208:string[])
              }
              event User Event {
                n105 = event-data() -> ("Workspace Event"=w222:string)  [unwired: 1 out]
                n106 = Equal?(x=w222, y="Shut Down") -> (x = y?=w223:bool)
                n107 = Equal?(x=w222, y="Disconnect") -> (x = y?=w224:bool)
                n108 = Compound Arithmetic op=OR(w223, w224) -> (w219:bool)
                n109 = case shown="True" w219 {
                  tunnel: [w229 w231] -> w221
                  tunnel: w220 -> [w229 w230]
                  frame False {
                  }
                  frame True {
                    n110 = Build Array (concatenate)(w230, "Object.Exit") -> (w231:string[])
                  }
                }
              }
              event User Event {
                # "Widget event has occurred.  Handle accordingly."
                n111 = event-data() -> ("ToWidgetMessage"=w238:T18)  [unwired: 1 out]
                n112 = case shown="Default" w238 {
                  tunnel: [w240 w243 w249] -> w237
                  tunnel: w236 -> [w240 w244 w250]
                  tunnel: w234 -> [w239 w241 w247]
                  tunnel: [w239 w241 w246] -> w233
                  frame Default {
                    # "Do nothing."
                  }
                  frame "Stop" {
                    # "User exiting workspace or deleting object"
                    n113 = Build Array (concatenate)(w244, "Object.Exit") -> (w243:string[])
                  }
                  frame "LaunchConfigDialog" {
                    # "User wants to configure object"
                    n114 = Build Array (concatenate)(w250, "Object.Configure") -> (w249:string[])
                    n115 = Bundle By Name(cluster=w247, "Data.PendingChange?"=FALSE ("Pending Change?")) -> (w246:T4)
                  }
                }
              }
              event Menu Selection (User) {
                n116 = event-data() -> ("ItemTag"=w253:string)  [unwired: 1 out]
                n117 = Build Array (concatenate)(w252, w253) -> (w251:string[])
              }
              event Panel Close? {
                n118 = event-data() -> ()  [unwired: 5 out]
                n119 = Build Array (concatenate)(w259, "Object.Exit") -> (w258:string[])
                n120 = event-data("Discard?"=TRUE) -> ()  [unwired: 1 in, 1 out]
              }
            }
          }
          frame "Object.Initialize" {
            # "Initialize the workspace Object state variables and UI"
            n121 = invoke on="DTCs" class="Tree (strict)" method="Edit Tree Items.Delete"(error in=w271, "Delete Children"=TRUE ("Delete Children?")) -> (error out=w266:errorcluster)  [unwired: 3 in, 4 out]
            n122 = local write "Tab Control"(0) -> ()
            n123 = Unbundle By Name(w267) -> ("UI.Refs.Filter Location"=w262:refnum<vi>, "UI.Refs.Override Byte Lengths"=w269:refnum<vi>)
            n124 = property class="Bool (strict)"(reference=w269, error in=w266, "Value"=FALSE) -> (error out=w264:errorcluster)  [unwired: 1 out]
            n125 = property class="Bool (strict)"(reference=w262, error in=w264, "Value"=FALSE) -> (error out=w263:errorcluster)  [unwired: 1 out]
          }
          frame "Object.Configure" {
            # "Allow the user to select a control object to display"
            n126 = Unbundle By Name(w281) -> ("NIVS.SysDefRoot"=w275:refnum<k24>, "CachedData.CD Path"=w282:string)
            n127 = call "Workspace.Select.Dialog.vi"("CD Path"=w282, "NIVS.System Definition Root"=w275) -> ("Cancelled?"=w279:bool, "IP Address"=w274:string, "Custom Device Path Out"=w278:string)  [unwired: 7 in]
            n128 = case shown="False" w279 {
              tunnel: w281 -> [w290 w291]
              tunnel: [w289 w291] -> w280
              tunnel: w278 -> [w288 _]
              tunnel: [w286 w292] -> w277
              tunnel: w276 -> [w287 w292]
              tunnel: w274 -> [w284 _]
              frame False {
                # "Queue up required states and cache new controller path"
                n129 = Bundle By Name(cluster=w290, "CachedData.CD Path"=w288, "CachedData.CD IP"=w284) -> (w289:T4)
                n130 = Build Array (concatenate)(w287, string[] ["Cache.Update", "Object.Initialize", "UI.Override.Hide", "VS.CheckConnect"]) -> (w286:string[])
              }
              frame True {
                # "User canceled"
              }
            }
          }
          frame "Object.Connected" {
            # "System state is Connected. Get path to required channels and start UDP acquisition if channels found."
            n131 = Unbundle By Name(w313) -> ("CachedData.CD Path"=w294:string, "NIVS.SysDefRoot"=w307:refnum<k24>, "UI.Refs.Cmd"=w305:refnum<vi>)
            n132 = call "UI.Addon.Path.Parse.vi"("Cached Addon Path"=w294) -> ("Addon Path"=w293:string)  [unwired: 6 in, 4 out]
            n133 = call "Workspace.Channels.Create.vi"("CD Path"=w294) -> ("Read Channels"=w311:string[], "Command Channel"=w310:string)  [unwired: 9 in]
            n134 = call "Workspace.CAN.Protocol.Get.vi"("error in (no error)"=w308, "Path"=w293, "NIVS.SysDef Ref"=w307) -> ("error out"=w309:errorcluster, "Diagnostic Protocol"=w306:T10)  [unwired: 7 in]
            n135 = case shown="\"User-Defined\"" w306 {
              tunnel: [w319 w321 w323] -> w304
              tunnel: [bool[] [TRUE, TRUE, TRUE] bool[] [TRUE, TRUE, TRUE] bool[] [TRUE, TRUE, FALSE]] -> w301
              frame "GMLAN" {
                w319 = T1[] [] items=["None", "Clear Status Channels", "Read All DIDs", "Read All PIDs", "Configure and Start DPIDs", "Stop DPIDs"] ("Disabled Items []")
              }
              frame "KWP-2000", "UDS" {
                w321 = T1[] [enum."Read All PIDs", enum."Configure and Start DPIDs", enum."Stop DPIDs"] items=["None", "Clear Status Channels", "Read All DIDs", "Read All PIDs", "Configure and Start DPIDs", "Stop DPIDs"] ("Disabled Items []")
              }
              frame "User-Defined" {
                w323 = T1[] [enum."Read All DIDs", enum."Read All PIDs", enum."Configure and Start DPIDs", enum."Stop DPIDs"] items=["None", "Clear Status Channels", "Read All DIDs", "Read All PIDs", "Configure and Start DPIDs", "Stop DPIDs"] ("Disabled Items []")
              }
            }
            n136 = Bundle By Name(cluster=w313, "Command.Channel"=w310, "Data.Read"=w311, "Diagnostic Protocol"=w306) -> (w296:T4)
            n137 = property class="Enum (strict)"(reference=w305, error in=w309, "Disabled Items []"=w304) -> (error out=w303:errorcluster)  [unwired: 1 out]
            n138 = property on="Tab Control" class="TabCtl (strict)"(error in=w303) -> (error out=w300:errorcluster, "Pages"=w302:refnum<vi>[])  [unwired: 1 in, 1 out]
            n139 = for {
              tunnel: w302 -> [w317] mode=indexing
              tunnel: w301 -> [w316] mode=indexing
              shift-right: [w314] -> w298
              shift-left: w300 -> [w315]
              n140 = property class="Page"(reference=w317, error in=w315, "PageVis"=w316) -> (error out=w314:errorcluster)  [unwired: 1 out]
            }
            n141 = call "Workspace.UI.DisableState.Set.vi"("Enable?"=TRUE, "error in (no error)"=w298, "State Variables in"=w296) -> ("error out"=w297:errorcluster, "State Variables out"=w295:T4)  [unwired: 7 in]
          }
          frame "Object.Disconnected" {
            n142 = call "Workspace.UI.DisableState.Set.vi"("Enable?"=FALSE, "error in (no error)"=w327, "State Variables in"=w326) -> ("error out"=w324:errorcluster, "State Variables out"=w325:T4)  [unwired: 7 in]
          }
          frame "VS.CheckConnect" {
            n143 = Unbundle By Name(w332) -> ("UI.Refs.Device"=w331:refnum<vi>, "NIVS.Workspace"=w343:T7, "NIVS.SysDefRoot"=w342:refnum<k24>, "CachedData.CD Path"=w341:string)
            n144 = Current VI's Menubar() -> (w344:refnum<k9>)
            n145 = call "UI.Connection.State.Get.vi"("Menu Ref"=w344, "Name Ref"=w331, "error in (no error)"=w340, "Addon Path in"=w341, "NIVS.System Definition Root in"=w342, "NIVS.Workspace Ref in"=w343) -> ("error out"=w339:errorcluster, "Addon Connected?"=w336:bool, "NIVS.System Definition Root out"=w337:refnum<k24>, "NIVS.Workspace Ref out"=w338:T7, "System Definition File"=w330:path)  [unwired: 1 in]
            n146 = case shown="False" w336 {
              tunnel: [w347 w350] -> w335
              tunnel: w334 -> [w346 w349]
              frame True {
                # "Addon connected"
                n147 = Build Array (concatenate)(w346, string[] ["Object.Connected", "Stream.Filter.Read"]) -> (w347:string[])
              }
              frame False {
                # "Addon not connected"
                n148 = Build Array (concatenate)(w349, string[] ["Object.Disconnected", "UI.Stream.Disabled", "Stream.Disable"]) -> (w350:string[])
              }
            }
            n149 = Bundle By Name(cluster=w332, "NIVS.SysDef"=w330, "NIVS.Workspace"=w338, "NIVS.SysDefRoot"=w337, "Addon.Connected?"=w336) -> (w333:T4)
          }
          frame "Object.Exit" {
            # "Stop current loop.  Queue Stop Acq and Exit to UDP loop."
            n150 = Unbundle By Name(w352) -> ("Stream.Qs"=w351:T11)
            n151 = call "Send Host Stream Command Exit.vi"("error in (no error)"=w353, "Q Refs"=w351) -> ("error out"=w354:errorcluster)  [unwired: 9 in]
          }
          frame "Cache.Update" {
            # "Cache any data needing to be permenantly stored with the workspace object."
            n152 = Unbundle By Name(w359) -> ("CachedData.UserEvent"=w357:refnum<user-event>, "CachedData"=w358:T6)
            n153 = Bundle By Name(cluster=T12 {"Operation"=enum."SetCustomData", "Data"=variant} ("event data"), "Data"=w358) -> (w360:T12)
            n154 = Generate User Event(user event=w357, event data cluster=w360) -> ()  [unwired: 2 in, 2 out]
          }
          frame "Channels.Get" {
            # "Get the current slow speed channel values from VeriStand if no pending change, data paths are valid and system state is connected."
            n155 = Unbundle By Name(w369) -> ("UI.Refs"=w364:T19, "Data.PendingChange?"=w365:bool, "Addon.Connected?"=w375:bool, "NIVS.Workspace"=w371:T7, "Data.Read"=w370:string[])  [unwired: 1 out]
            n156 = case shown="False" w375 {
              tunnel: w374 -> [w382 w388]
              tunnel: [w382 w387] -> w366
              tunnel: w371 -> [w381 w386]
              tunnel: [w381 w385] -> w368
              tunnel: w370 -> [w380 w384]
              tunnel: [w377 w383] -> w367
              frame False {
                # "Do Nothing."
                n157 = Array Size(array=w380) -> (size(s)=w379:i32)
                n158 = Initialize Array(0.0 ("element"), w379) -> (w377:dbl[])
              }
              frame True {
                # "Connected & paths valid"
                n159 = call-poly <vilib>:"NI VeriStand - Get Channel Value.vi"("error in (no error)"=w388, "Channels"=w384, "WorkspaceManager in"=w386) -> ("error out"=w387:errorcluster, "Values"=w383:dbl[], "WorkspaceManager out"=w385:T7)  [unwired: 6 in]
              }
            }
            n160 = call "Workspace.UI.Update.vi"("error in (no error)"=w366, "Data.PendingChange?"=w365, "Values"=w367, "UI.Refs"=w364) -> ("error out"=w373:errorcluster)  [unwired: 7 in]
            n161 = Bundle By Name(cluster=w369, "NIVS.Workspace"=w368, "Data.PreviousValues"=w367) -> (w372:T4)
          }
          frame "Channels.Set" {
            # "Set Channels if data paths are valid and system state is connected and there is a change in the data value."
            n162 = Unbundle By Name(w396) -> ("Addon.Connected?"=w392:bool, "NIVS.Workspace"=w391:T7, "Command.Channel"=w389:string, "UI.Refs"=w390:T19)
            n163 = case shown="False" w392 {
              tunnel: w398 -> [w401 w403]
              tunnel: [w401 w409] -> w397
              tunnel: w391 -> [w400 w408]
              tunnel: [w400 w407] -> w393
              tunnel: w389 -> [_ w406]
              tunnel: w390 -> [_ w404]
              frame False {
                # "Do nothing"
              }
              frame True {
                # "Connected & paths valid"
                n164 = call "Workspace.UI.Pull.vi"("error in (no error)"=w403, "UI.Refs"=w404) -> ("error out"=w402:errorcluster, "Value"=w405:dbl)  [unwired: 8 in]
                n165 = call-poly <vilib>:"NI VeriStand - Set Channel Value.vi"("error in (no error)"=w402, "Value"=w405, "Channel"=w406, "WorkspaceManager in"=w408) -> ("error out"=w409:errorcluster, "WorkspaceManager out"=w407:T7)  [unwired: 6 in]
              }
            }
            n166 = Bundle By Name(cluster=w396, "Data.PendingChange?"=FALSE ("Pending Change?"), "NIVS.Workspace"=w393) -> (w395:T4)
          }
          frame "UI.Override.Hide" {
            # "Reset slow speed channel displayed values."
            n167 = Unbundle By Name(w416) -> ("UI.Refs.DTC"=w415:refnum<vi>, "UI.Refs.Status"=w414:refnum<vi>, "UI.Refs.Failure"=w413:refnum<vi>)
            n168 = Build Array(w415, w414, w413) -> (w412:refnum<vi>[])
            n169 = for {
              tunnel: w412 -> [w422] mode=indexing
              shift-right: [w420] -> w410
              shift-left: w411 -> [w421]
              n170 = property class="DigNum (strict)"(reference=w422, error in=w421, "Visible"=FALSE, "Value"=u32 0) -> (error out=w420:errorcluster)  [unwired: 1 out]
            }
          }
          frame "UI.Override.Show" {
            # "Reset slow speed channel displayed values."
            n171 = Unbundle By Name(w429) -> ("UI.Refs.DTC"=w428:refnum<vi>, "UI.Refs.Status"=w427:refnum<vi>, "UI.Refs.Failure"=w426:refnum<vi>)
            n172 = Build Array(w428, w427, w426) -> (w425:refnum<vi>[])
            n173 = for {
              tunnel: w425 -> [w434] mode=indexing
              shift-right: [w432] -> w423
              shift-left: w424 -> [w433]
              n174 = property class="DigNum (strict)"(reference=w434, error in=w433, "Visible"=TRUE) -> (error out=w432:errorcluster)  [unwired: 1 out]
            }
          }
          frame "UI.Stream.Enabled" {
            n175 = call "UI.Stream.Enable.vi"("error in (no error)"=w436, "State Variables in"=w435) -> ("error out"=w437:errorcluster)  [unwired: 9 in]
          }
          frame "UI.Log.Enabled" {
            w439 = T20."Disabled and Grayed Out" ("Disabled")
            n176 = Unbundle By Name(w451) -> ("UI.Refs.Type Filter"=w444:refnum<vi>, "UI.Refs.Filter IDs"=w443:refnum<vi>, "UI.Refs.Direction Filter"=w442:refnum<vi>, "UI.Refs.Reset Filter"=w447:refnum<vi>, "UI.Refs.Filter Location"=w450:refnum<vi>)
            n177 = property class="Bool (strict)"(reference=w450, error in=w449, "DisabledEnum"=w439) -> (error out=w448:errorcluster, "Value"=w446:bool)  [unwired: 1 out]
            n178 = Build Array(w444, w443, w442) -> (w441:refnum<vi>[])
            n179 = property class="Bool"(reference=w447, error in=w448, "DisabledEnum"=w439) -> (error out=w445:errorcluster)  [unwired: 1 out]
            n180 = case shown="False" w446 {
              tunnel: w445 -> [w455 w461]
              tunnel: w441 -> [w456 _]
              tunnel: [w454 w461] -> w440
              tunnel: w439 -> [w453 _]
              frame False {
                n181 = for {
                  tunnel: w456 -> [w460] mode=indexing
                  shift-right: [w458] -> w454
                  shift-left: w455 -> [w459]
                  tunnel: w453 -> [w457]
                  n182 = property class="Ctl"(reference=w460, error in=w459, "DisabledEnum"=w457) -> (error out=w458:errorcluster)  [unwired: 1 out]
                }
              }
              frame True {
              }
            }
          }
          frame "UI.Stream.Disabled" {
            n183 = call "UI.Stream.Disable.vi"("error in (no error)"=w463, "State Variables in"=w464) -> ("error out"=w462:errorcluster)  [unwired: 9 in]
          }
          frame "UI.Log.Disabled" {
            w466 = T20."Enabled" ("Disabled")
            n184 = Unbundle By Name(w477) -> ("UI.Refs.Type Filter"=w471:refnum<vi>, "UI.Refs.Filter IDs"=w470:refnum<vi>, "UI.Refs.Direction Filter"=w469:refnum<vi>, "UI.Refs.Reset Filter"=w473:refnum<vi>, "UI.Refs.Filter Location"=w476:refnum<vi>)
            n185 = property class="Bool (strict)"(reference=w476, error in=w475, "DisabledEnum"=w466) -> (error out=w474:errorcluster)  [unwired: 1 out]
            n186 = Build Array(w471, w470, w469) -> (w468:refnum<vi>[])
            n187 = property class="Bool"(reference=w473, error in=w474, "DisabledEnum"=w466) -> (error out=w472:errorcluster)  [unwired: 1 out]
            n188 = for {
              tunnel: w468 -> [w482] mode=indexing
              shift-right: [w480] -> w467
              shift-left: w472 -> [w481]
              tunnel: w466 -> [w479]
              n189 = property class="Ctl"(reference=w482, error in=w481, "DisabledEnum"=w479) -> (error out=w480:errorcluster)  [unwired: 1 out]
            }
          }
          frame "Raw.Send" {
            # "Reset slow speed channel displayed values."
            n190 = Unbundle By Name(w497) -> ("CachedData.CD IP"=w486:string, "CachedData.CD Path"=w484:string)
            n191 = call "UI.Addon.Path.Parse.vi"("Cached Addon Path"=w484) -> ("Addon Name"=w483:string)  [unwired: 6 in, 4 out]
            n192 = Bundle By Name(cluster=cluster{"cmd":u8[], "require response?":bool} {"cmd"=[], "require response?"=TRUE} ("Cmd"), "cmd"="Raw Cmd", "require response?"="Response Required?") -> (w495:cluster{"cmd":u8[], "require response?":bool})
            n193 = call "Connect.vi"("Addon Name"=w483, "Address"=w486) -> ("error out"=w492:errorcluster, "Ref"=w498:T21)  [unwired: 8 in]
            n194 = call "PassThru.vi"("error in (no error)"=w492, "timeout ms (1000)"=2500, "Cmd"=w495, "Ref"=w498) -> ("error out"=w491:errorcluster, "Resp"=w490:T25, "Ref"=w499:T21)  [unwired: 5 in]
            n195 = Unbundle By Name(w490) -> ("resp"=→"Raw Resp":u8[], "error code"=→"Raw Error Byte":u8, "error out"=→"Raw VeriStand Error":errorcluster)
            n196 = call "Disconnect.vi"("error in"=w491, "Ref"=w499) -> ()  [unwired: 9 in, 1 out]
          }
          frame "Raw.Clear" {
            n197 = local write "Raw Cmd"(u8[] [] ("Cmd")) -> ()
          }
          frame "DTC.Read" {
            # "Reset slow speed channel displayed values."
            n198 = Unbundle By Name(w529) -> ("CachedData.CD IP"=w527:string, "CachedData.CD Path"=w528:string)
            n199 = Bundle By Name(cluster=T13 {"Extension"=0, "Mask"=0, "Mode/Status"=0, "Byte Lengths"={"Override"=FALSE, "DTC"=0, "Status"=0, "Failure"=0}} ("Options (KWP/UDS Only)"), "Extension"="Extension", "Mask"="Mask", "Mode/Status"="Mode", "Byte Lengths.Override"="Override Byte Lengths", "Byte Lengths.DTC"="DTC", "Byte Lengths.Status"="Status", "Byte Lengths.Failure"="Failure") -> (w521:T13)
            n200 = call "UI.Addon.Path.Parse.vi"("Cached Addon Path"=w528) -> ("Addon Name"=w506:string)  [unwired: 6 in, 4 out]
            n201 = call "Connect.vi"("Addon Name"=w506, "Address"=w527) -> ("error out"=w525:errorcluster, "Ref"=w526:T21)  [unwired: 8 in]
            n202 = call "ReadDTCs.vi"("error in (no error)"=w525, "timeout ms (1000)"=2500, "Options (KWP/UDS Only)"=w521, "Ref"=w526) -> ("error out"=w524:errorcluster, "Active DTCs"=w511:T26[], "Ref"=w523:T21)  [unwired: 5 in]
            n203 = call "Disconnect.vi"("error in"=w524, "Ref"=w523) -> ("error out"=w516:errorcluster)  [unwired: 9 in]
            n204 = control-ref of="DTCs"() -> (w508:refnum<vi>)
            n205 = call <vilib>:"Simple Error Handler.vi"("error in (no error)"=w516) -> ()  [unwired: 4 in, 5 out]
            n206 = call "Workspace.DTC.Update.vi"("Hex"="Hex", "error in"=w509, "Active DTCs"=w511, "DTCs"=w508) -> ("error out"=w507:errorcluster)  [unwired: 7 in]
          }
          frame "Stream.Enable" {
            n207 = Unbundle By Name(w536) -> ("Stream.Qs"=w533:T11, "CachedData.CD IP"=w534:string, "CachedData.CD Path"=w540:string, "NIVS.SysDef"=w532:path)
            n208 = Strip Path(path=w532) -> (stripped path=w531:path)  [unwired: 1 out]
            n209 = call "UI.Addon.Path.Parse.vi"("Cached Addon Path"=w540) -> ("Addon Name"=w535:string)  [unwired: 6 in, 4 out]
            n210 = call "Send Host Stream Command Start.vi"("Project Folder"=w531, "error in (no error)"=w538, "Addon"=w535, "Target IP Address"=w534, "Q Refs"=w533) -> ("error out"=w537:errorcluster)  [unwired: 6 in]
          }
          frame "Stream.Filter.Send" {
            n211 = Unbundle By Name(w553) -> ("CachedData.CD IP"=w551:string, "CachedData.CD Path"=w554:string)
            n212 = local read "Direction Filter"() -> (w542:T3)
            n213 = local read "Type Filter"() -> (w543:T2)
            n214 = local read "Filter IDs"() -> (w544:string)
            n215 = call "Convert Filter IDs String to Array.vi"("Filter IDs"=w544) -> ("Filter IDs"=w541:u32[])  [unwired: 10 in]
            n216 = call "UI.Addon.Path.Parse.vi"("Cached Addon Path"=w554) -> ("Addon Name"=w552:string)  [unwired: 6 in, 4 out]
            n217 = Bundle By Name(cluster=T15 {"ID Filters"=[], "Direction Filter"=enum."Tx/Rx", "Type Filter"=enum."All"} ("IDs"), "Direction Filter"=w542, "Type Filter"=w543, "ID Filters"=w541) -> (w545:T15)
            n218 = call "Connect.vi"("Addon Name"=w552, "Address"=w551) -> ("error out"=w548:errorcluster, "Ref"=w547:T21)  [unwired: 8 in]
            n219 = call "SetStreamingFilter.vi"("error in (no error)"=w548, "IDs"=w545, "Ref"=w547) -> ("error out"=w556:errorcluster, "Ref"=w555:T21)  [unwired: 7 in]
            n220 = call "Disconnect.vi"("error in"=w556, "Ref"=w555) -> ("error out"=w549:errorcluster)  [unwired: 9 in]
            n221 = call <vilib>:"Simple Error Handler.vi"("error in (no error)"=w549) -> ()  [unwired: 4 in, 5 out]
          }
          frame "Stream.Filter.Clear" {
            n222 = Unbundle By Name(w565) -> ("CachedData.CD IP"=w563:string, "CachedData.CD Path"=w566:string)
            n223 = call "UI.Addon.Path.Parse.vi"("Cached Addon Path"=w566) -> ("Addon Name"=w564:string)  [unwired: 6 in, 4 out]
            n224 = call "Connect.vi"("Addon Name"=w564, "Address"=w563) -> ("error out"=w560:errorcluster, "Ref"=w559:T21)  [unwired: 8 in]
            n225 = call "SetStreamingFilter.vi"("error in (no error)"=w560, "IDs"=T15 {"ID Filters"=[], "Direction Filter"=enum."Tx/Rx", "Type Filter"=enum."All"}, "Ref"=w559) -> ("error out"=w568:errorcluster, "Ref"=w567:T21)  [unwired: 7 in]
            n226 = call "Disconnect.vi"("error in"=w568, "Ref"=w567) -> ("error out"=w561:errorcluster)  [unwired: 9 in]
            n227 = call <vilib>:"Simple Error Handler.vi"("error in (no error)"=w561) -> ()  [unwired: 4 in, 5 out]
          }
          frame "Stream.Filter.Reset" {
            n228 = Unbundle By Name(w582) -> ("CachedData.CD IP"=w580:string, "CachedData.CD Path"=w583:string)
            n229 = call "UI.Addon.Path.Parse.vi"("Cached Addon Path"=w583) -> ("Addon Name"=w581:string)  [unwired: 6 in, 4 out]
            n230 = call "Connect.vi"("Addon Name"=w581, "Address"=w580) -> ("error out"=w577:errorcluster, "Ref"=w576:T21)  [unwired: 8 in]
            n231 = call "ResetStreamingFilter.vi"("error in (no error)"=w577, "Ref"=w576) -> ("error out"=w585:errorcluster, "IDs"=w572:T15, "Ref"=w584:T21)  [unwired: 7 in]
            n232 = local write "Host Filter"(FALSE ("Host Filter")) -> ()
            n233 = Unbundle By Name(w572) -> ("ID Filters"=w571:u32[], "Direction Filter"=w574:T3, "Type Filter"=w573:T2)
            n234 = call "Disconnect.vi"("error in"=w585, "Ref"=w584) -> ("error out"=w578:errorcluster)  [unwired: 9 in]
            n235 = call <vilib>:"Simple Error Handler.vi"("error in (no error)"=w578) -> ()  [unwired: 4 in, 5 out]
            n236 = call "Convert Filter IDs Array to String.vi"("Filter IDs"=w571) -> ("Filter IDs"=w570:string)  [unwired: 10 in]
            n237 = local write "Filter IDs"(w570) -> ()
            n238 = local write "Direction Filter"(w574) -> ()
            n239 = local write "Type Filter"(w573) -> ()
          }
          frame "Stream.Filter.Read" {
            n240 = Unbundle By Name(w599) -> ("CachedData.CD IP"=w597:string, "CachedData.CD Path"=w600:string)
            n241 = call "UI.Addon.Path.Parse.vi"("Cached Addon Path"=w600) -> ("Addon Name"=w598:string)  [unwired: 6 in, 4 out]
            n242 = call "Connect.vi"("Addon Name"=w598, "Address"=w597) -> ("error out"=w603:errorcluster, "Ref"=w604:T21)  [unwired: 8 in]
            n243 = call "GetStreamingFilter.vi"("error in (no error)"=w603, "Ref"=w604) -> ("error out"=w602:errorcluster, "IDs"=w594:T15, "Ref"=w601:T21)  [unwired: 7 in]
            n244 = Unbundle By Name(w594) -> ("ID Filters"=w591:u32[], "Direction Filter"=w593:T3, "Type Filter"=w592:T2)
            n245 = call "Disconnect.vi"("error in"=w602, "Ref"=w601) -> ("error out"=w595:errorcluster)  [unwired: 9 in]
            n246 = call <vilib>:"Simple Error Handler.vi"("error in (no error)"=w595) -> ()  [unwired: 4 in, 5 out]
            n247 = local write "Direction Filter"(w593) -> ()
            n248 = local write "Type Filter"(w592) -> ()
            n249 = Array To Spreadsheet String(delimiter (Tab)=",", array=w591, 3:"x%x" ("format string")) -> (spreadsheet string=w588:string)
            n250 = call <vilib>:"Trim Whitespace.vi"("string"=w588) -> ("trimmed string"=w587:string)  [unwired: 1 in]
            n251 = local write "Filter IDs"(w587) -> ()
          }
          frame "Stream.Table.GoUp" {
            n252 = Unbundle By Name(w610) -> ("UI.Refs.Table Control"=w608:refnum<vi>)
            n253 = property class="Tbl (strict)"(reference=w608, error in=w606, "Index Values"=T16 {"Row"=0, "Column"=0}) -> (error out=w607:errorcluster)  [unwired: 1 out]
          }
          frame "Stream.Disable" {
            n254 = Unbundle By Name(w615) -> ("Stream.Qs"=w614:T11)
            n255 = call "Send Host Stream Command Stop.vi"("error in (no error)"=w612, "Q Refs"=w614) -> ("error out"=w613:errorcluster)  [unwired: 9 in]
          }
        }
      }
      frame Error {
        # "Handle Errors."
        n256 = Unbundle By Name(w619) -> ("code"=w623:i32)
        n257 = Equal?(x=-307654, y=w623) -> (x = y?=w621:bool)
        n258 = Select(t=errorcluster {"status"=FALSE, "code"=0, "source"=""}, s=w621, f=w619) -> (s? t:f=w618:errorcluster)
        n259 = call <vilib>:"Simple Error Handler.vi"("error in (no error)"=w618) -> ("error out"=w624:errorcluster)  [unwired: 4 in, 4 out]
        n260 = call <vilib>:"Clear Errors.vi"("error in (no error)"=w624) -> ("error out"=w617:errorcluster)  [unwired: 5 in, 1 out]
      }
    }
  }
  n261 = while {
    tunnel: w10 -> [w653]
    tunnel: w9 -> [w652]
    tunnel: [w645] -> w8
    stop <- w644 stop-if-true
    n262 = Unbundle By Name(w652) -> ("UI.Refs.CAN State"=w649:refnum<vi>, "Stream.Qs"=w651:T11)
    n263 = call "Convert Filter IDs String to Array.vi"("Filter IDs"="Filter IDs") -> ("Filter IDs"=w627:u32[])  [unwired: 10 in]
    n264 = Bundle By Name(cluster=T27 {"Host Filter"=FALSE, "Filter Parameters"={"ID Filters"=[], "Direction Filter"=enum."Tx/Rx", "Type Filter"=enum."All"}, "Sort By ID"=FALSE, "Pause"=FALSE, "Clear History"=FALSE, "Log"=FALSE} ("Host Parameters"), "Clear History"="Clear History", "Pause"="Pause", "Sort By ID"="Sort By ID", "Filter Parameters.Direction Filter"="Direction Filter", "Filter Parameters.Type Filter"="Type Filter", "Host Filter"="Host Filter", "Log"="Log", "Filter Parameters.ID Filters"=w627) -> (w639:T27)
    n265 = call "Main Engine Host Stream.vi"("error in (no error)"=w653, "Host Parameters"=w639, "Q Refs"=w651) -> ("error out"=w650:errorcluster, "Exit"=w644:bool, "Stream"=w648:T28)  [unwired: 6 in]
    n266 = Unbundle By Name(w648) -> ("Bus Warning"=w647:bool, "Connected"=→"Stream Connected":bool, "Bus Status"=w638:string, "Log Status"=w634:string, "Bus Data Update"=w633:bool, "Bus Data"=w632:string[][])
    n267 = property class="Str"(reference=w649, error in=w650, "Blinking"=w647) -> (error out=w645:errorcluster)  [unwired: 1 out]
    n268 = Concatenate Strings(w638, "\r\n", w634) -> (→"Status":string)
    n269 = case shown="True" w633 {
      tunnel: w632 -> [_ w654]
      frame False {
      }
      frame True {
        "Table Control" <- w654
      }
    }
  }
  n270 = flat-sequence {
    tunnel: w36 -> [w655]
    tunnel: w8 -> [_]
    frame #0 {
      n271 = call "Workspace.Close.vi"("State Variables in"=w655) -> ()  [unwired: 11 in]
    }
    frame #1 {
      n272 = invoke class="VI" method="FP.Close"() -> ()  [unwired: 3 in, 3 out]
    }
  }
